vi "CSM - Read INI String.vi"(5 "Section Name(\"\" as Default)":string, 7 "error in (no error)":errorcluster, 9 "String in":string) -> (1 "error out":errorcluster, 2 "Key Found?":bool, 3 "String out":string)   [LabVIEW 2017, in "INI-Static-Variable-Support.lvlib"]
uses:
  _Support/_fgv-oper.ctl
  _Support/global-csm-ini-db-change-flag.vi
  INI-Static-Variable-Support.lvlib
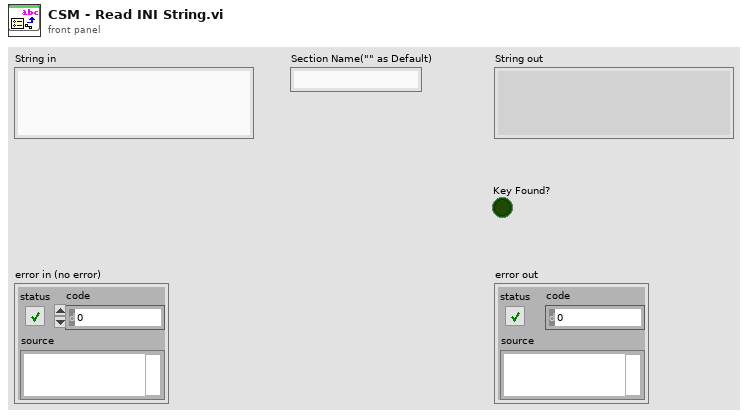
[diagram p1: front panel]
types:
  T1 = typedef "_fgv-oper.ctl" = enum16{"Read", "Write", "Sync"}
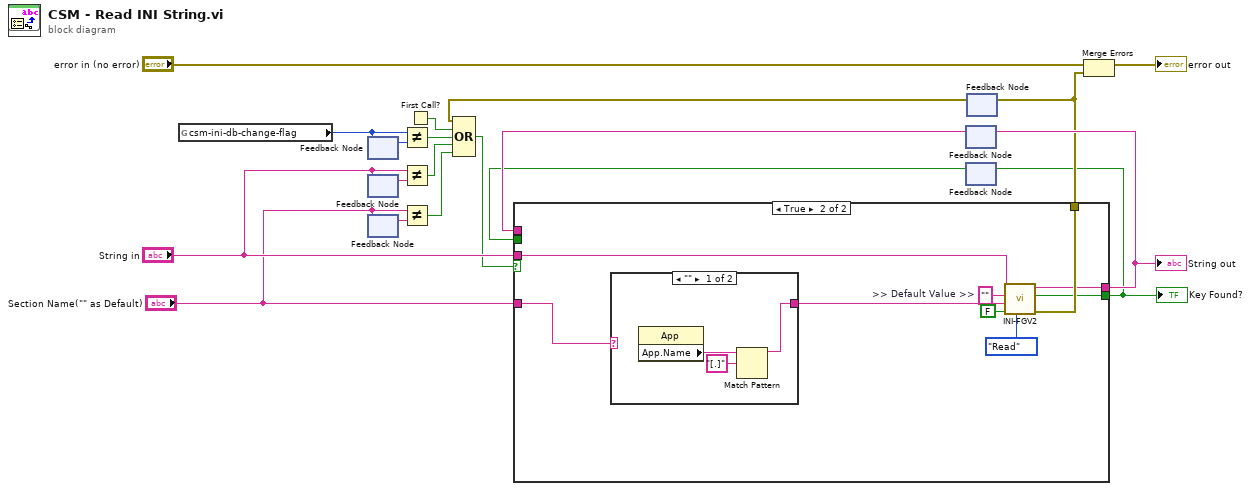
[diagram p0: block diagram]
diagram:
  n1 = global read "global-csm-ini-db-change-flag.vi" "csm-ini-db-change-flag"() -> (w17:u32)
  n2 = feedback #1() -> (w16:u32)  [unwired: 1 in]
  n3 = feedback-in #1(w17) -> ()
  n4 = feedback #2() -> (w13:string)  [unwired: 1 in]
  n5 = feedback-in #2("String in") -> ()
  n6 = feedback #3() -> (w12:string)  [unwired: 1 in]
  n7 = feedback-in #3("Section Name(\"\" as Default)") -> ()
  n8 = Not Equal?(x=w17, y=w16) -> (x != y?=w15:bool)
  n9 = Not Equal?(x="String in", y=w13) -> (x != y?=w9:bool)
  n10 = Not Equal?(x="Section Name(\"\" as Default)", y=w12) -> (x != y?=w8:bool)
  n11 = First Call?() -> (First Call?: T/F=w14:bool)
  n12 = feedback #4() -> (w6:string)  [unwired: 1 in]
  n13 = feedback #5() -> (w3:bool)  [unwired: 1 in]
  n14 = feedback #6() -> (w2:errorcluster)  [unwired: 1 in]
  n15 = Compound Arithmetic op=OR(w2, w14, w15, w9, w8) -> (w1:bool)
  n16 = case shown="True" w1 {
    tunnel: [_ w27] -> w5
    tunnel: [w21 w26] -> w7
    tunnel: [w20 w25] -> w4
    tunnel: "String in" -> [_ w24]
    tunnel: "Section Name(\"\" as Default)" -> [_ w23]
    tunnel: w6 -> [w21 _]
    tunnel: w3 -> [w20 _]
    frame False {
    }
    frame True {
      w28 = ""  # >> Default Value >>
      n17 = case shown="\"\"" w23 {
        selector: w23 -> [_ w34]
        tunnel: [w31 w34] -> w22
        frame "" {
          n18 = property class="App"() -> ("App.Name"=w32:string)  [unwired: 2 in, 2 out]
          n19 = Match Pattern(string=w32, regular expression="[.]") -> (before substring=w31:string)  [unwired: 1 in, 3 out]
        }
        frame Default {
        }
      }
      n20 = call "INI-FGV2.vi"("Enum"=_fgv-oper."Read", "Raw String? (F)"=FALSE, ">> Section >>"=w22, ">> Default Value >>"=w28, ">> Variable Name >>"=w24) -> ("error out"=w27:errorcluster, "Key?"=w25:bool, "Value"=w26:string)  [unwired: 4 in]
    }
  }
  "String out" <- w7
  "Key Found?" <- w4
  n21 = feedback-in #4(w7) -> ()
  n22 = feedback-in #5(w4) -> ()
  n23 = feedback-in #6(w5) -> ()
  n24 = Merge Errors("error in (no error)", w5) -> (→"error out":errorcluster)
